vi "robot_efg_choose_step.vi"(8 "error In":errorcluster, 9 "JSON string":string, 10 "Step order":string, 11 "process_ID":string) -> (0 "error IO":errorcluster)   [LabVIEW 2020]
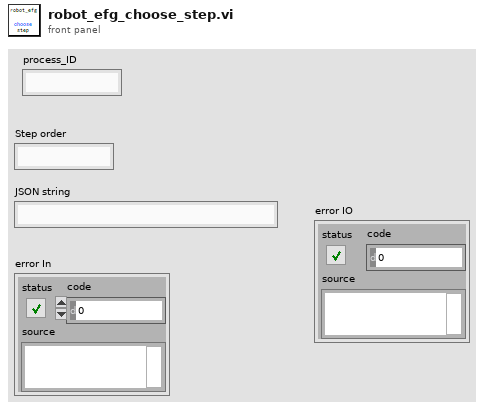
[diagram p1: front panel]
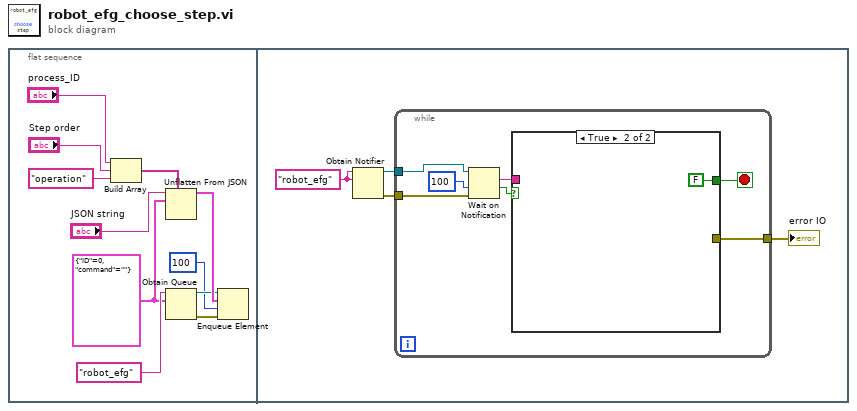
[diagram p0: block diagram]
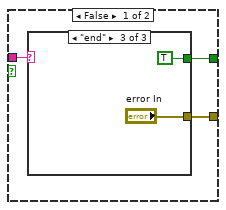
[diagram p2: hidden frame]
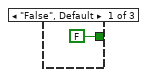
[diagram p3: hidden frame]
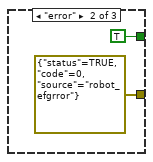
[diagram p4: hidden frame]
diagram:
  n1 = flat-sequence {
    frame #0 {
      w1 = cluster{"ID":i32, "command":string} {"ID"=0, "command"=""} ("参数")
      n2 = Build Array("process_ID", "Step order", "operation" ("string")) -> (w8:string[])
      n3 = Unflatten From JSON(path=w8, JSON string="JSON string", type and defaults=w1) -> (value=w11:cluster{"ID":i32, "command":string})  [unwired: 4 in, 1 out]
      n4 = Obtain Queue(name (unnamed)="robot_efg", element data type=w1) -> (queue out=w9:refnum<queue>, error out=w10:errorcluster)  [unwired: 3 in, 1 out]
      n5 = Enqueue Element(queue=w9, element=w11, timeout in ms (-1)=100, error in (no error)=w10) -> ()  [unwired: 3 out]
    }
    frame #1 {
      w12 = "robot_efg" ("name (unnamed)")
      n6 = Obtain Notifier(name (unnamed)=w12, notification data type=w12) -> (notifier out=w15:refnum<notifier>, error out=w14:errorcluster)  [unwired: 2 in, 1 out]
      n7 = while {
        tunnel: w15 -> [w22]
        tunnel: w14 -> [w19]
        tunnel: [w16] -> w13
        stop <- w17 stop-if-true
        n8 = Wait on Notification(notifier=w22, timeout in ms (-1)=100, error in (no error)=w19) -> (notification=w18:string, timed out?=w20:bool)  [unwired: 1 in, 2 out]
        n9 = case shown="True" w20 {
          tunnel: w18 -> [w25 _]
          tunnel: [w24 FALSE] -> w17
          tunnel: [w23 _] -> w16
          frame False {
            n10 = case shown="\"end\"" w25 {
              tunnel: [FALSE TRUE TRUE] -> w24
              tunnel: [_ errorcluster {"status"=TRUE, "code"=0, "source"="robot_efgrror"} ("error IO") "error In"] -> w23
              frame "False", Default {
              }
              frame "error" {
              }
              frame "end" {
              }
            }
          }
          frame True {
          }
        }
      }
      "error IO" <- w13
    }
  }
